vi "CheckBounceStatus.vi"(0 "Parameters in":T1={"bounce?"=FALSE, "black?"=FALSE, "slide number"=-1, "hide?"=FALSE, "selection"=FALSE}, 1 "File Name":string) -> (2 "Parameters":T1, 3 "With parameters":string, 4 "file name":string)   [LabVIEW 2014]
uses:
  ParamterCluster.ctl
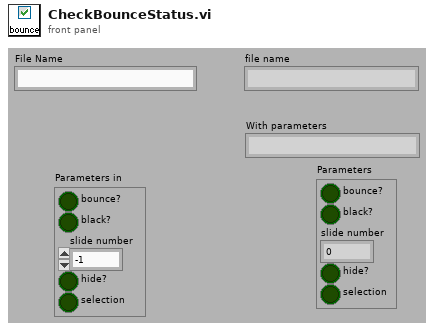
[diagram p1: front panel]
types:
  T1 = typedef "ParamterCluster.ctl" = cluster{"bounce?":bool, "black?":bool, "slide number":i32, "hide?":bool, "selection":bool}
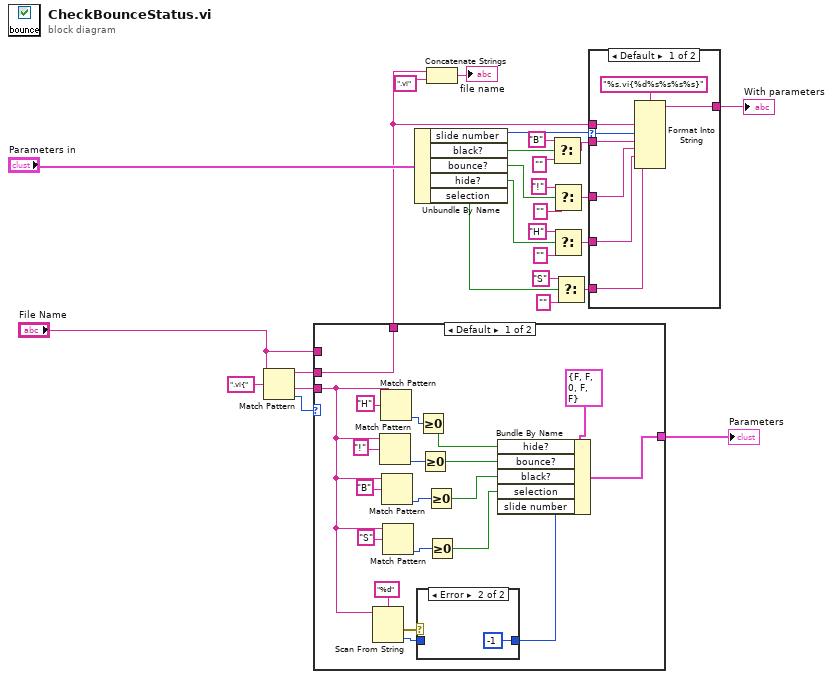
[diagram p0: block diagram]
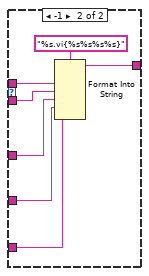
[diagram p2: hidden frame]
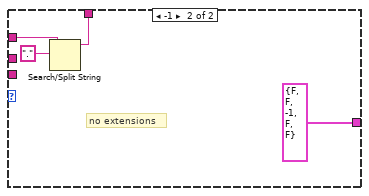
[diagram p4: hidden frame]
diagram:
  n1 = Match Pattern(string="File Name", regular expression=".vi{") -> (before substring=w15:string, after substring=w25:string, offset past match=w28:i32)  [unwired: 1 in, 1 out]
  n2 = case shown="Default" w28 {
    tunnel: [w37 T1 {"bounce?"=FALSE, "black?"=FALSE, "slide number"=-1, "hide?"=FALSE, "selection"=FALSE} ("Parameters")] -> w26
    tunnel: w25 -> [w31 _]
    tunnel: [w36 w51] -> w2
    tunnel: w15 -> [w36 _]
    tunnel: "File Name" -> [_ w53]
    frame Default {
      n3 = Scan From String(format string="%d", input string=w31) -> (error out=w40:errorcluster, output 1=w38:i32)  [unwired: 3 in, 2 out]
      n4 = Match Pattern(string=w31, regular expression="!") -> (offset past match=w46:i32)  [unwired: 1 in, 3 out]
      n5 = Match Pattern(string=w31, regular expression="H") -> (offset past match=w34:i32)  [unwired: 1 in, 3 out]
      n6 = Match Pattern(string=w31, regular expression="B") -> (offset past match=w44:i32)  [unwired: 1 in, 3 out]
      n7 = Match Pattern(string=w31, regular expression="S") -> (offset past match=w32:i32)  [unwired: 1 in, 3 out]
      n8 = case shown="Error" w40 {
        tunnel: [w49 -1] -> w39
        tunnel: w38 -> [w49 _]
        frame No Error {
        }
        frame Error {
        }
      }
      n9 = Greater Or Equal To 0?(x=w34) -> (x >= 0?=w33:bool)
      n10 = Greater Or Equal To 0?(x=w46) -> (x >= 0?=w45:bool)
      n11 = Greater Or Equal To 0?(x=w44) -> (x >= 0?=w42:bool)
      n12 = Greater Or Equal To 0?(x=w32) -> (x >= 0?=w29:bool)
      n13 = Bundle By Name(cluster=T1 {"bounce?"=FALSE, "black?"=FALSE, "slide number"=0, "hide?"=FALSE, "selection"=FALSE} ("Parameters"), "hide?"=w33, "bounce?"=w45, "black?"=w42, "selection"=w29, "slide number"=w39) -> (w37:T1)
    }
    frame -1 {
      # "no extensions"
      n14 = Search/Split String(string=w53, search string/char (-)="." ("regular expression")) -> (substring before match=w51:string)  [unwired: 1 in, 2 out]
    }
  }
  "Parameters" <- w26
  n15 = Unbundle By Name("Parameters in") -> ("slide number"=w1:i32, "black?"=w24:bool, "bounce?"=w20:bool, "hide?"=w9:bool, "selection"=w4:bool)
  n16 = Concatenate Strings(w2, ".vi" ("regular expression")) -> (→"file name":string)
  n17 = Select(t="B" ("format string"), s=w24, f="" ("format string")) -> (s? t:f=w21:string)
  n18 = Select(t="!" ("format string"), s=w20, f="" ("format string")) -> (s? t:f=w17:string)
  n19 = Select(t="H" ("format string"), s=w9, f="" ("format string")) -> (s? t:f=w7:string)
  n20 = Select(t="S" ("format string"), s=w4, f="" ("format string")) -> (s? t:f=w3:string)
  n21 = case shown="Default" w1 {
    selector: w1 -> [w55 _]
    tunnel: w21 -> [w62 w63]
    tunnel: w17 -> [w61 w69]
    tunnel: [w59 w67] -> w13
    tunnel: w7 -> [w58 w66]
    tunnel: w3 -> [w57 w65]
    tunnel: w2 -> [w56 w64]
    frame Default {
      n22 = Format Into String(format string="%s.vi{%d%s%s%s%s}", w56, w55, w62, w61, w58, w57) -> (resulting string=w59:string)  [unwired: 2 in, 1 out]
    }
    frame -1 {
      n23 = Format Into String(format string="%s.vi{%s%s%s%s}", w64, w63, w69, w66, w65) -> (resulting string=w67:string)  [unwired: 2 in, 1 out]
    }
  }
  "With parameters" <- w13
